vi "Drive_SetMotorsSpeed.vi"(7 "ControlMode":T5, 8 "error in":errorcluster, 9 "Right_Speed":dbl, 10 "Left_Speed":dbl, 11 "CAN Jaguars Ref":T1) -> (0 "error out":errorcluster, 3 "CAN Jaguars Ref out":T1)   [LabVIEW 2009, in "Drive.lvlib"]
doc: "This VI sets speed for left and right motor. Speed range is -1..+1, where -1 is full reverse speed, +1 - full forward speed."
uses:
  Drive.lvlib
  Drive_ControlMode.ctl
  OWNCAN/CAN Jaguars Ref.ctl
  CAN/SubVIs/CAN Jaguar Ref.ctl
  CAN/SubVIs/CAN Jaguar Control Mode.ctl
  PWM/PWM_Name.ctl
  Motor.lvlib
  PWM.lvlib
  OWNCAN.lvlib
  CAN.lvlib
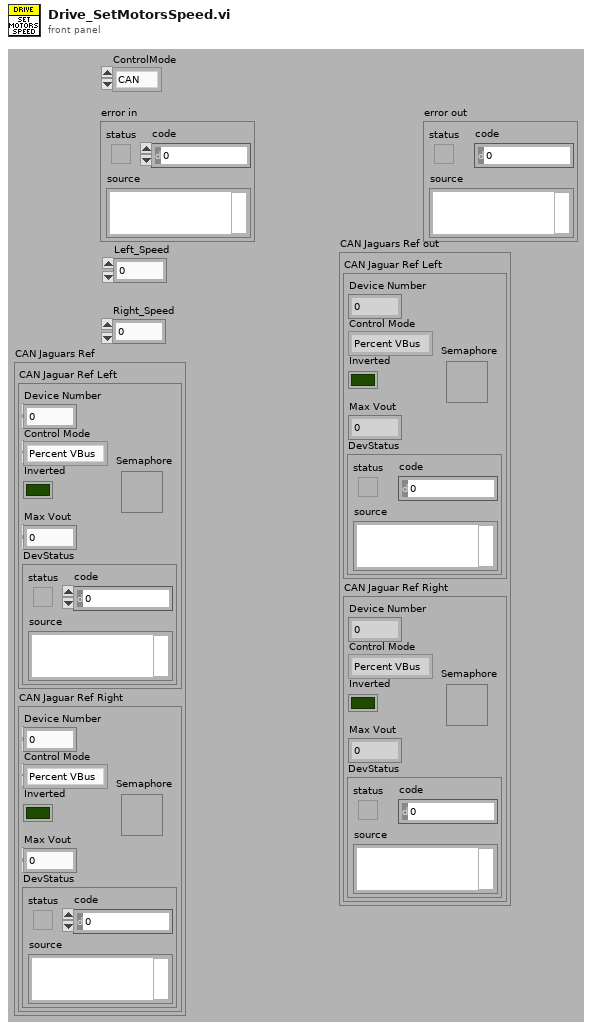
[diagram p1: front panel]
types:
  T1 = typedef "OWNCAN.lvlib/CAN Jaguars Ref.ctl" = cluster{"CAN Jaguar Ref Left":T2, "CAN Jaguar Ref Right":T2}
  T2 = typedef "CAN.lvlib/CAN Jaguar Ref.ctl" = cluster{"Device Number":u8, "Control Mode":T3, "Inverted":bool, "Semaphore":T4, "Max Vout":dbl, "DevStatus":errorcluster}
  T3 = typedef "CAN.lvlib/CAN Jaguar Control Mode.ctl" = enum16{"Percent VBus", "Speed", "Position", "Current"}
  T4 = typedef "Semaphore RefNum" = refnum<k1>
  T5 = typedef "Drive.lvlib/Drive_ControlMode.ctl" = enum16{"CAN", "PWM"}
  T6 = typedef "PWM.lvlib/PWM_Name.ctl" = u16
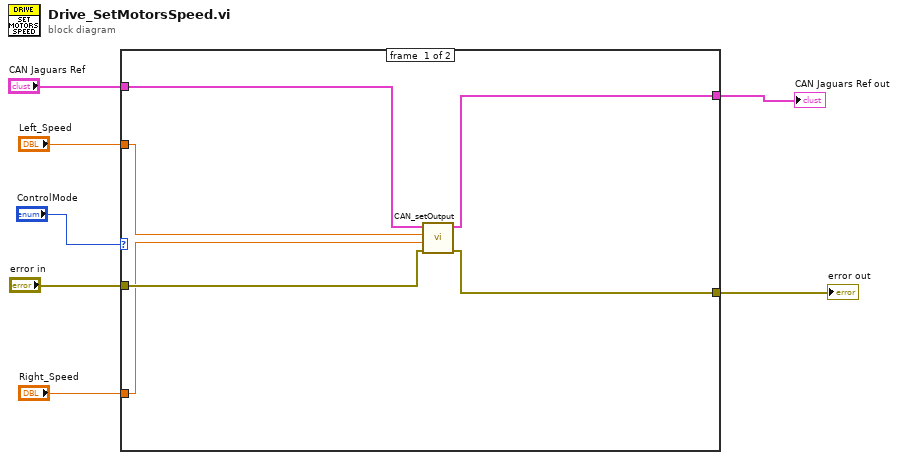
[diagram p0: block diagram]
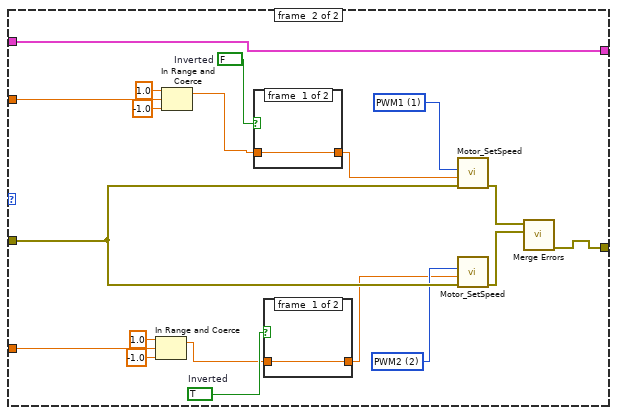
[diagram p2: hidden frame]
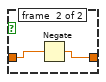
[diagram p3: hidden frame]
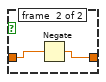
[diagram p4: hidden frame]
diagram:
  n1 = case shown="\"PWM\"" "ControlMode" {
    tunnel: [w12 w32] -> w7
    tunnel: "error in" -> [w13 w29]
    tunnel: "Left_Speed" -> [w10 w28]
    tunnel: "Right_Speed" -> [w11 w25]
    tunnel: "CAN Jaguars Ref" -> [w9 w14]
    tunnel: [w8 w14] -> w1
    frame #0 {
      n2 = call "CAN_setOutput.vi"("error in (no error)"=w13, "Output Right"=w11, "Output Left"=w10, "CAN Jaguars Ref"=w9) -> ("error out"=w12:errorcluster, "CAN Jaguars Ref out"=w8:T1)  [unwired: 6 in]
    }
    frame #1 {
      w17 = TRUE  # Inverted
      w18 = FALSE  # Inverted
      w21 = T6 2 items=["Invalid"=0, "PWM1"=1, "PWM2"=2, "PWM9"=9, "PWM10"=10] ("PWM_Channel")
      w22 = T6 1 items=["Invalid"=0, "PWM1"=1, "PWM2"=2, "PWM9"=9, "PWM10"=10] ("PWM_Channel")
      n3 = In Range and Coerce(upper limit=1.0, x=w25, lower limit=-1.0) -> (coerced(x)=w15:dbl)  [unwired: 1 out]
      n4 = In Range and Coerce(upper limit=1.0, x=w28, lower limit=-1.0) -> (coerced(x)=w20:dbl)  [unwired: 1 out]
      n5 = case shown="True" w18 {
        tunnel: w20 -> [w36 w37]
        tunnel: [w36 w38] -> w19
        frame #0 {
        }
        frame #1 {
          n6 = Negate(x=w37) -> (-x=w38:dbl)
        }
      }
      n7 = case shown="False" w17 {
        tunnel: w15 -> [w33 w34]
        tunnel: [w33 w35] -> w16
        frame #0 {
        }
        frame #1 {
          n8 = Negate(x=w34) -> (-x=w35:dbl)
        }
      }
      n9 = call "Motor_SetSpeed.vi"("error in"=w29, "Speed"=w19, "PWM_Channel"=w22) -> ("error out"=w31:errorcluster)  [unwired: 8 in]
      n10 = call "Motor_SetSpeed.vi"("error in"=w29, "Speed"=w16, "PWM_Channel"=w21) -> ("error out"=w30:errorcluster)  [unwired: 8 in]
      n11 = call <vilib>:"Merge Errors.vi"("error in 2 (no error)"=w30, "error in 1 (no error)"=w31) -> ("error out"=w32:errorcluster)  [unwired: 5 in]
    }
  }
  "error out" <- w7
  "CAN Jaguars Ref out" <- w1
